vi "GenNet Add Broadcast Name To Variant.vi"(10 "Broadcast Name":string, 11 "Broadcast Data IN":variant) -> (3 "Variant OUT":variant)   [LabVIEW 2014, in "hse-gennet.lvlib"]
uses:
  hse-gennet.lvlib
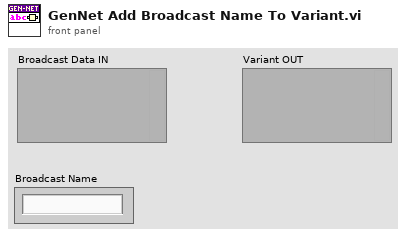
[diagram p1: front panel]
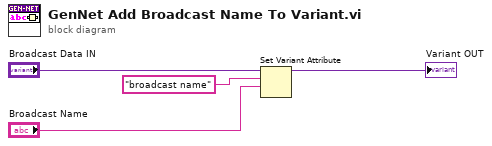
[diagram p0: block diagram]
diagram:
  n1 = Set Variant Attribute(Variant="Broadcast Data IN", name="broadcast name", value="Broadcast Name") -> (Variant out=→"Variant OUT":variant)  [unwired: 1 in, 2 out]
